vi "INDEXING PATH (SubVI).vi"(10 "ORDER ID:-":dbl, 11 "ROWS":string[](array[string])) -> (1 "STRING":string, 2 "PRODUCT AVAILABLITY":bool=TRUE, 3 "INDIDCATOR":bool)   [LabVIEW 2020]
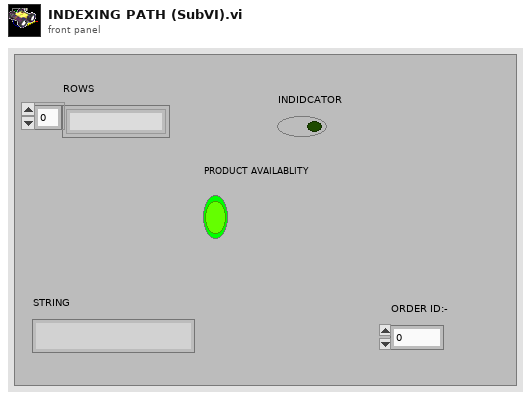
[diagram p1: front panel]
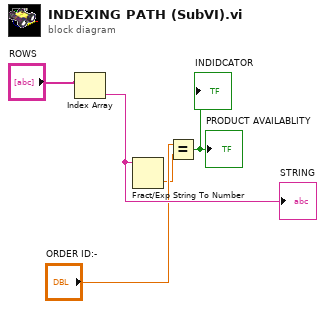
[diagram p0: block diagram]
diagram:
  n1 = Index Array(array="ROWS") -> (element=w3:string)  [unwired: 1 in]
  "STRING" <- w3
  n2 = Fract/Exp String To Number(string=w3) -> (number=w1:dbl)  [unwired: 3 in, 1 out]
  n3 = Equal?(x="ORDER ID:-", y=w1) -> (x = y?=→"PRODUCT AVAILABLITY" →"INDIDCATOR":bool)
